vi "HSDIO_6541_Session_Init.vi"(8 "error in (no error)":errorcluster, 10 "Use Software Trigger":bool=TRUE, 11 "HSDIO 6541 Inputs":T1={"Resource Name"="Sequencer", "Clock Rate"=1000000.0, "Trigger Source"="PFI0"} {"Clock Rate" format="%.2p"}) -> (0 "error out":errorcluster, 3 "instrument handle out":refnum<k15>)   [LabVIEW 2015]
doc: "This VI inits a waveform generation session for HSDIO 6541. This is a basic example that shows how to setup the board in order to generate waveforms according to a script. \n\n1. Initialize for a generation session.\n2. Assign specified channels in Channel List for dynamic operation : all = \"\" (default)\n3. Sets the Idle State for when the generation has completed : NO !!\n4. Configure the Sample clock to use the onboard clock, and configure the clock rate.\n5. Set generation mode to Scripted.\n6. Configure the Script Trigger : change to Digital Edge if waiting for an external\n trigger, and link Rising Edge and source trigger commands.\n Use PFI0 with SMB wired to the board, or any PFIxx if connected to accessory."
uses:
  controls/HSDIO_6541_Inputs.ctl
  <instrlib>/niHSDIO/niHSDIO.llb/niHSDIO_ctl Trigger Source Values (Ring).ctl
  <instrlib>/niHSDIO/niHSDIO.llb/niHSDIO_ctl Generation Mode Values (Ring).ctl
  <instrlib>/niHSDIO/niHSDIO.llb/niHSDIO_ctl Sample Clock Source Values (ComboBox).ctl
  <instrlib>/niHSDIO/niHSDIO.llb/niHSDIO_ctl Trigger DigEdge - Edge Values (Ring).ctl
  <instrlib>/niHSDIO/niHSDIO.llb/niHSDIO_ctl Trigger Script - trigID Values (Ring).ctl
  <instrlib>/niHSDIO/niHSDIO.llb/niHSDIO Configure Digital Edge Script Trigger.vi
  <instrlib>/niHSDIO/niHSDIO.llb/niHSDIO Configure Software Script Trigger.vi
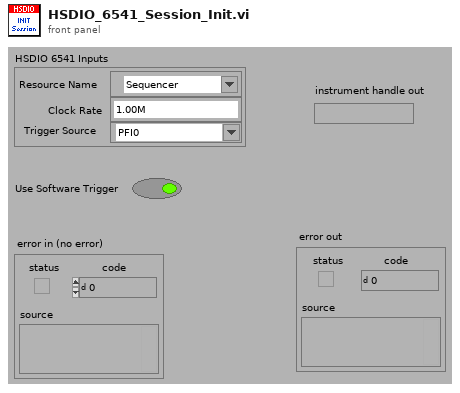
[diagram p1: front panel]
types:
  T1 = typedef "HSDIO_6541_Inputs.ctl" = cluster{"Resource Name":refnum<k15>, "Clock Rate":dbl, "Trigger Source":T2}
  T2 = typedef "niHSDIO_ctl Trigger Source Values (Ring).ctl" = string
  T3 = typedef "niHSDIO_ctl Sample Clock Source Values (ComboBox).ctl" = string
  T4 = typedef "niHSDIO_ctl Generation Mode Values (Ring).ctl" = i32
  T5 = typedef "niHSDIO_ctl Trigger Script - trigID Values (Ring).ctl" = string
  T6 = typedef "niHSDIO_ctl Trigger DigEdge - Edge Values (Ring).ctl" = i32
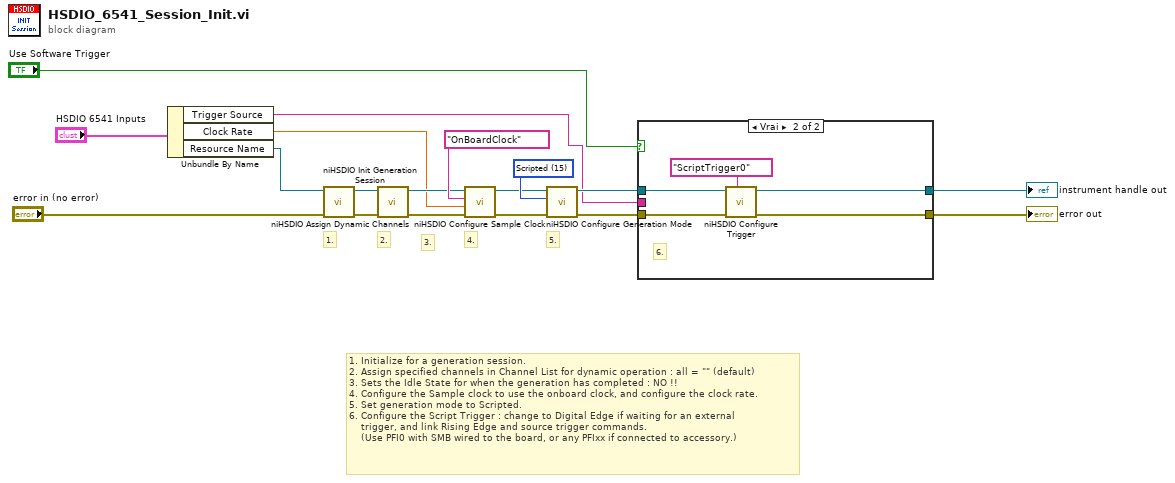
[diagram p0: block diagram]
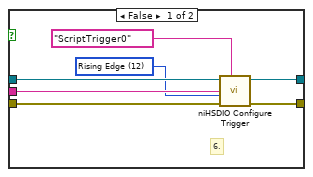
[diagram p2: hidden frame]
diagram:
  w11 = T4 15 items=["Waveform"=14, "Scripted"=15] ("generation mode (waveform)")
  # "5."
  # "4."
  # "3."
  # "2."
  # "1."
  # "1. Initialize for a generation session.\n2. Assign specified channels in Channel List for dynamic operation : all = \"\" (default)\n3. Sets the Idle State for when the generation has completed : NO !!\n4. Configure the Sample clock to use the onboard clock, and configure the clock rate.\n5. Set generation mode to Scripted.\n6. Configure the Script Trigger : change to Digital Edge if waiting for an external\n    trigger, and link Rising Edge and source trigger commands.\n    (Use PFI0 with SMB wired to the board, or any PFIxx if connected to accessory.)"
  n1 = Unbundle By Name("HSDIO 6541 Inputs") -> ("Trigger Source"=w3:T2, "Clock Rate"=w4:dbl, "Resource Name"=w2:refnum<k15>)
  n2 = call <instrlib>:"niHSDIO Init Generation Session.vi"("error in (no error)"="error in (no error)", "resource name"=w2) -> ("error out"=w13:errorcluster, "instrument handle out"=w14:refnum<k15>)  [unwired: 8 in]
  n3 = call <instrlib>:"niHSDIO Assign Dynamic Channels.vi"("error in (no error)"=w13, "instrument handle"=w14) -> ("error out"=w7:errorcluster, "instrument handle out"=w8:refnum<k15>)  [unwired: 8 in]
  n4 = call <instrlib>:"niHSDIO Configure Sample Clock.vi"("error in (no error)"=w7, "clock rate (50MHz)"=w4, "clock source (on board clock)"=T3 "OnBoardClock", "instrument handle"=w8) -> ("error out"=w9:errorcluster, "instrument handle out"=w10:refnum<k15>)  [unwired: 6 in]
  n5 = call <instrlib>:"niHSDIO Configure Generation Mode.vi"("error in (no error)"=w9, "generation mode (waveform)"=w11, "instrument handle"=w10) -> ("error out"=w5:errorcluster, "instrument handle out"=w6:refnum<k15>)  [unwired: 7 in]
  n6 = case shown="Vrai" "Use Software Trigger" {
    tunnel: w6 -> [w25 w30]
    tunnel: w5 -> [w24 w29]
    tunnel: [w23 w28] -> w18
    tunnel: [w22 w27] -> w17
    tunnel: w3 -> [w21 _]
    frame False {
      w20 = T6 12 items=["Rising Edge"=12, "Falling Edge"=13] ("Edge")
      # "6."
      n7 = call-poly <instrlib>:"niHSDIO Configure Trigger.vi"("trigger id (script trigger 0)"=T5 "ScriptTrigger0", "error in (no error)"=w24, "edge (rising)"=w20, "source (PFI 0)"=w21, "instrument handle"=w25) -> ("error out"=w22:errorcluster, "instrument handle out"=w23:refnum<k15>)  [unwired: 5 in]
    }
    frame True {
      # "6."
      n8 = call-poly <instrlib>:"niHSDIO Configure Trigger.vi"("trigger id (script trigger 0)"=T5 "ScriptTrigger0", "error in (no error)"=w29, "instrument handle"=w30) -> ("error out"=w27:errorcluster, "instrument handle out"=w28:refnum<k15>)  [unwired: 7 in]
    }
  }
  "instrument handle out" <- w18
  "error out" <- w17
